vi "SCM1 Empty Buffer.vi"(2 "error in (no error)":errorcluster, 3 "VISA Resource Name":refnum<visa-resource-name>) -> (0 "error out":errorcluster, 1 "dup VISA Resource Name":refnum<visa-resource-name>)   [LabVIEW 2024]
panel:
  out "Array":string[](array[string])
  out "Numeric":i32
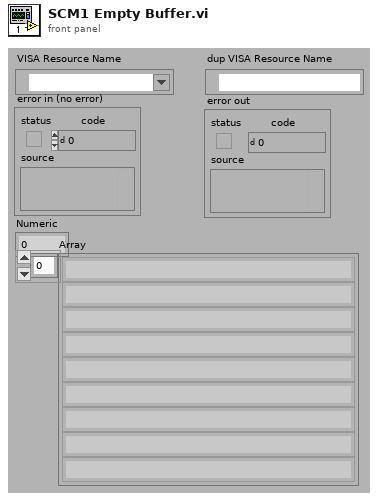
[diagram p1: front panel]
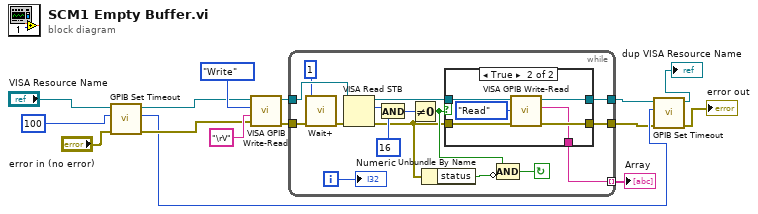
[diagram p0: block diagram]
diagram:
  n1 = call "GPIB Set Timeout.vi"("Error In"="error in (no error)", "Timeout"=u32 100 ("General Settings:Timeout Value"), "VISA resource name"="VISA Resource Name") -> ("Error Out"=w8:errorcluster, "Old Timeout"=w4:u32, "dup VISA resource name"=w11:refnum<visa-resource-name>)  [unwired: 2 in]
  n2 = call "VISA GPIB Write-Read.vi"("error in (no error)"=w8, "Command"="\rV" ("String to Write"), "Action"=enum16{"Write", "Read", "Write & Read"}."Write", "VISA resource name"=w11) -> ("error out"=w13:errorcluster, "dup VISA Session"=w12:refnum<visa-resource-name>)  [unwired: 4 in, 2 out]
  n3 = while {
    tunnel: w12 -> [w19]
    tunnel: w13 -> [w17]
    tunnel: [w23] -> w2
    tunnel: [w22] -> w3
    tunnel: [w20] -> w10 mode=indexing
    i -> [w21]
    stop <- w26 continue-if-true
    n4 = call "Wait+.vi"("Error In"=w17, "milliseconds to wait"=u32 1) -> ("Error Out"=w16:errorcluster)  [unwired: 4 in, 1 out]
    n5 = VISA Read STB(8:w16, 11:w19) -> (0:w25:errorcluster, 2:w31:u16, 3:w28:refnum<visa-resource-name>)
    n6 = And(x=w31, y=u16 16) -> (x .and. y?=w29:u16)
    n7 = Not Equal To 0?(x=w29) -> (x != 0?=w27:bool)
    n8 = Unbundle By Name(w25) -> ("status"=w24:bool)
    n9 = case shown="True" w27 {
      tunnel: w25 -> [w32 w38]
      tunnel: w28 -> [w33 w37]
      tunnel: [w32 w36] -> w23
      tunnel: [w33 w35] -> w22
      tunnel: [_ w34] -> w20
      frame False {
      }
      frame True {
        n10 = call "VISA GPIB Write-Read.vi"("error in (no error)"=w38, "Action"=enum16{"Write", "Read", "Write & Read"}."Read", "VISA resource name"=w37) -> ("error out"=w36:errorcluster, "String Returned"=w34:string, "dup VISA Session"=w35:refnum<visa-resource-name>)  [unwired: 5 in, 1 out]
      }
    }
    n11 = Compound Arithmetic op=AND(w27, invert w24) -> (w26:bool)
    "Numeric" <- w21
  }
  "Array" <- w10
  n12 = call "GPIB Set Timeout.vi"("Error In"=w2, "Timeout"=w4, "VISA resource name"=w3) -> ("Error Out"=→"error out":errorcluster, "dup VISA resource name"=→"dup VISA Resource Name":refnum<visa-resource-name>)  [unwired: 2 in, 1 out]
